vi "Format Error Response.vi"(7 "show call chain? (False)":bool, 8 "error in (no error)":errorcluster, 11 "Error Response":string) -> (0 "error out":errorcluster)   [LabVIEW 2023, in "CTI-Visa.lvlib"]
uses:
  CTI-Visa.lvlib
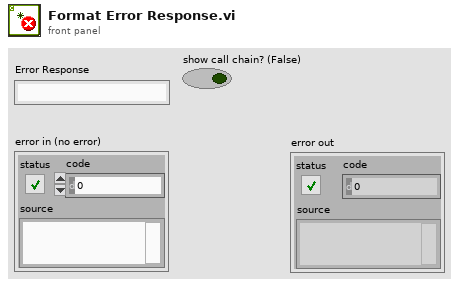
[diagram p1: front panel]
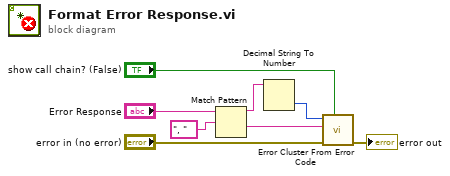
[diagram p0: block diagram]
diagram:
  n1 = Match Pattern(string="Error Response", regular expression=", " ("x")) -> (before substring=w6:string, after substring=w4:string)  [unwired: 1 in, 2 out]
  n2 = Decimal String To Number(string=w6) -> (number=w5:i32)  [unwired: 2 in, 1 out]
  n3 = call <vilib>:"Error Cluster From Error Code.vi"("show call chain? (False)"="show call chain? (False)", "error in (no error)"="error in (no error)", "error message (\"\")"=w4, "error code (0)"=w5) -> ("error out"=→"error out":errorcluster)  [unwired: 5 in]
